vi "CRYConvertResultWorkin.vi"(6 "Work in":u16, 7 "Type":u16(slide) caption="Type:", 8 "unit":string, 9 "IsTrue":bool, 10 "Margin In":dbl) -> (1 "Margin Out":dbl)   [LabVIEW 2013]
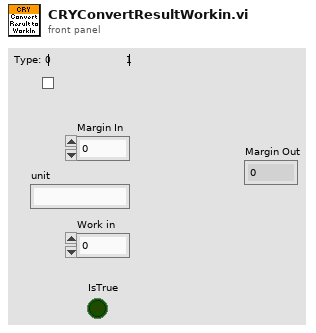
[diagram p1: front panel]
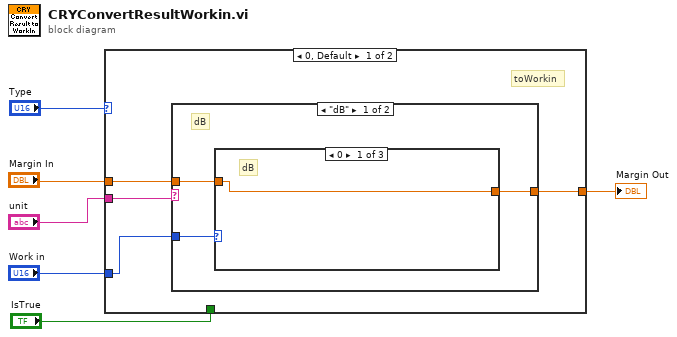
[diagram p0: block diagram]
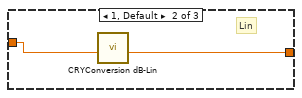
[diagram p2: hidden frame]
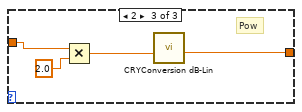
[diagram p3: hidden frame]
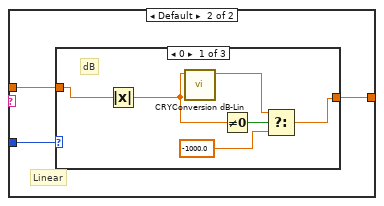
[diagram p4: hidden frame]
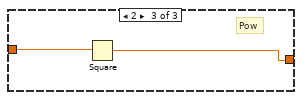
[diagram p6: hidden frame]
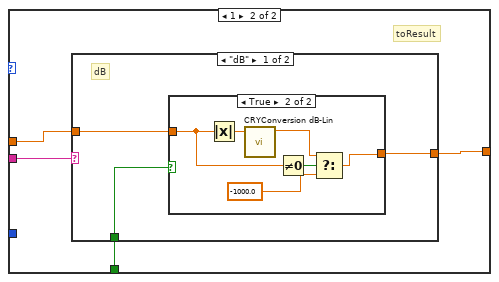
[diagram p7: hidden frame]
diagram:
  n1 = case shown="0, Default" "Type" {
    tunnel: "Margin In" -> [w8 w35]
    tunnel: "Work in" -> [w9 _]
    tunnel: "unit" -> [w10 w36]
    tunnel: [w7 w34] -> w2
    tunnel: "IsTrue" -> [_ w33]
    frame 0, Default {
      # "toWorkin"
      n2 = case shown="\"dB\"" w10 {
        tunnel: [w11 w21] -> w7
        tunnel: w9 -> [w13 w23]
        tunnel: w8 -> [w12 w22]
        frame "dB" {
          # "dB"
          n3 = case shown="0" w13 {
            tunnel: w12 -> [w14 w16 w19]
            tunnel: [w14 w15 w20] -> w11
            frame 0 {
              # "dB"
            }
            frame 1, Default {
              # "Lin"
              n4 = call "CRYConversion dB-Lin.vi"("Log In"=w16) -> ("Lin Out"=w15:dbl)  [unwired: 5 in, 3 out]
            }
            frame 2 {
              # "Pow"
              n5 = Multiply(x=w19, y=2.0) -> (x*y=w17:dbl)
              n6 = call "CRYConversion dB-Lin.vi"("Log In"=w17) -> ("Lin Out"=w20:dbl)  [unwired: 5 in, 3 out]
            }
          }
        }
        frame Default {
          # "Linear"
          n7 = case shown="0" w23 {
            tunnel: w22 -> [w29 w30 w32]
            tunnel: [w24 w30 w31] -> w21
            frame 0 {
              # "dB"
              n8 = Absolute Value(x=w29) -> (abs(x)=w28:dbl)
              n9 = call "CRYConversion dB-Lin.vi"("Lin In"=w28) -> ("Log Out"=w26:dbl)  [unwired: 5 in, 3 out]
              n10 = Not Equal To 0?(x=w28) -> (x != 0?=w27:bool)
              n11 = Select(t=w26, s=w27, f=-1000.0) -> (s? t:f=w24:dbl)
            }
            frame 1, Default {
              # "Lin"
            }
            frame 2 {
              # "Pow"
              n12 = Square(x=w32) -> (x^2=w31:dbl)
            }
          }
        }
      }
    }
    frame 1 {
      # "toResult"
      n13 = case shown="\"dB\"" w36 {
        tunnel: [w38 w47] -> w34
        tunnel: w35 -> [w39 w47]
        tunnel: w33 -> [w37 _]
        frame "dB" {
          # "dB"
          n14 = case shown="True" w37 {
            tunnel: w39 -> [w40 w43]
            tunnel: [w40 w42] -> w38
            frame False {
            }
            frame True {
              n15 = Absolute Value(x=w43) -> (abs(x)=w46:dbl)
              n16 = call "CRYConversion dB-Lin.vi"("Lin In"=w46) -> ("Log Out"=w41:dbl)  [unwired: 5 in, 3 out]
              n17 = Not Equal To 0?(x=w43) -> (x != 0?=w44:bool)
              n18 = Select(t=w41, s=w44, f=-1000.0) -> (s? t:f=w42:dbl)
            }
          }
        }
        frame Default {
          # "Linear"
        }
      }
    }
  }
  "Margin Out" <- w2
